vi "Volume data viewer tool.vi"() -> ()   [LabVIEW 2017]
uses:
  <vilib>/addons/Biomedical/NI_BMTK_Controls.lvlib
  <vilib>/addons/Biomedical/Controls/Medical Image/Medical Image 2D Viewer Helper (2D U16).vi
  Typedefs/Save-Load enum.ctl
  <vilib>/addons/Biomedical/Controls/Medical Image/2D Image Viewer/Medical Image 2D Viewer.xctl
panel:
  out "2D Viewer":i32[][][](xcontrol)
  in  "Selected Plane":i32(slide) scale=1.0..5.0
  in  "TDMS file path & name":path=path "C:/Users/Theo/Desktop/Volume Acquisition/Volume acquisition TDMS data files/001.tdms"
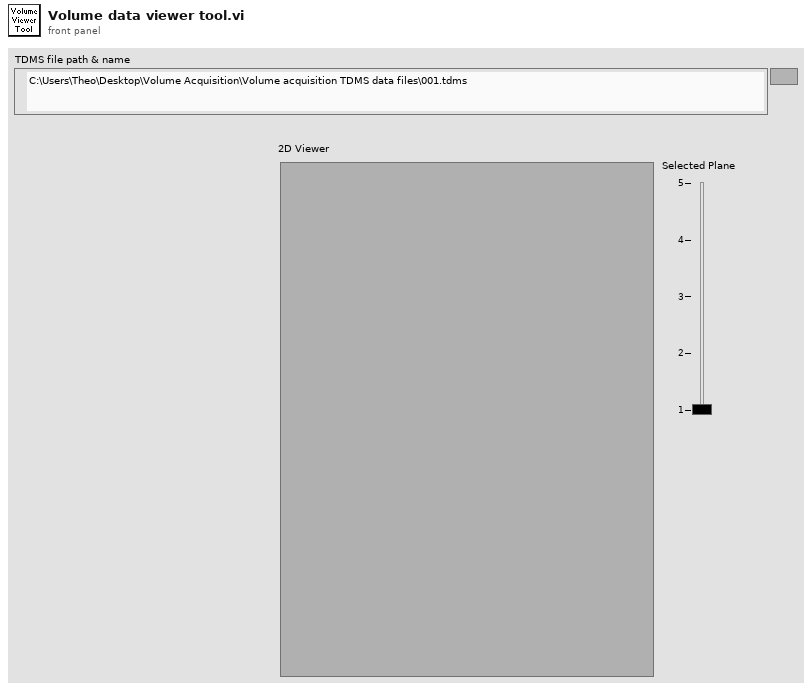
[diagram p1: front panel]
types:
  T1 = typedef "Save-Load enum.ctl" = enum16{"Save to file", "Load from file", "Compare from file"}
  T2 = typedef "Header parameters cluster-ALL.ctl" = cluster{"Imaging Protocol":T3, "Number of POI":u16, "Number of Miniscans":u16, "Number of Trials":u16, "Number of Cycles ":u64, "# Averaged Frames":u16, "Laser power (%)":u8, "Pockels":dbl, "Acquisition Length (sec)":dbl, "Fill time (us)":dbl, "POI Dwell time (us)":dbl, "Miniscan Dwell time per pixel (us)":dbl, "PMT 1":dbl, "PMT 2":dbl, "Back Apperture":dbl, "Zoom":dbl, "Frame Size":T4, "Center Frequency":dbl, "Field of View":dbl, "DwellTime (us)":dbl, "Wavelength (nm)":dbl, "AOL Z":dbl, "AOL Mode":T5, "GridXY":dbl, "GridZ":dbl, "TriggerDelay (sec)":dbl, "Number of Pixels in Miniscan":u16, "Experiment folder path":path, "X centre":dbl, "Y centre":dbl, "Angle (degrees)":dbl, "Plane Mode":T6, "Software version":dbl, "Objective":T7, "MotorZ Calibration":u32, "Pockels Calibration":u32, "Threshold":u16[], "Video length (sec)":dbl, "Frame rate (fps)":u8, "Rectangle ROI length (pixels)":u16, "Rectangle ROI height (pixels)":u16}
  T3 = typedef "Imaging Protocols enum.ctl" = enum16{"AOL Z-Stack", "Motor Z Stack", "Functional Acquisition", "Single Plane Acquisition", "Volume Acquisition", "Live Imaging", "Live Plane Imaging", "Live Volume Imaging"}
  T4 = typedef "Frame Size.ctl" = u16
  T5 = typedef "AOL modes.ctl" = enum16{"Raster", "Structural", "Pointing", "Mini Scan", "Alignment"}
  T6 = typedef "Plane Mode.ctl" = u16
  T7 = typedef "Objective selector control enum.ctl" = string
  T8 = cluster{"Number of cycles":i32, "number of planes":i32, "number of miniscans in a Plane":i32, "number of pixels in a miniscan":i32}
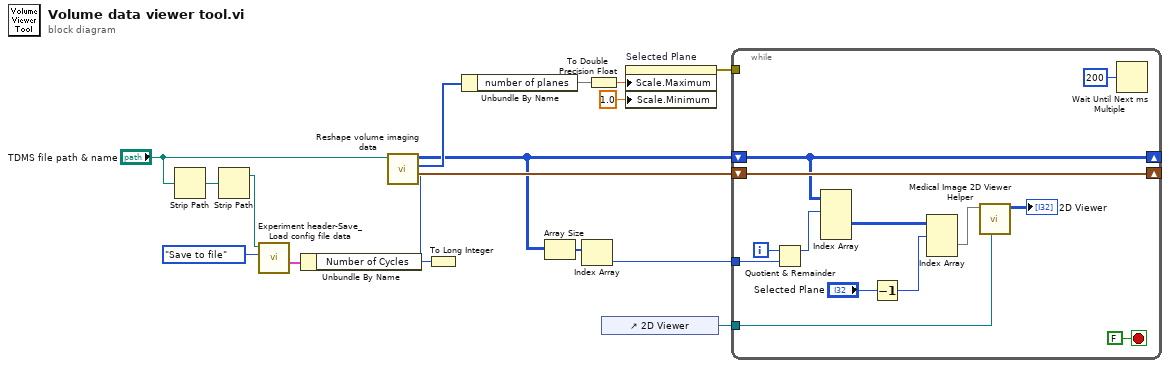
[diagram p0: block diagram]
diagram:
  n1 = Strip Path(path="TDMS file path & name") -> (stripped path=w5:path)  [unwired: 1 out]
  n2 = Strip Path(path=w5) -> (stripped path=w3:path)  [unwired: 1 out]
  n3 = call "Experiment header-Save_Load config file data.vi"("Function"=Save-Load_enum."Save to file", "Experiment data folder path"=w3) -> ("All header parameters out"=w6:T2)  [unwired: 8 in, 1 out]
  n4 = Unbundle By Name(w6) -> ("Number of Cycles"=w2:u64)
  n5 = To Long Integer(number=w2) -> (32bit integer=w1:i32)
  n6 = call "Reshape volume imaging data.vi"(9:w1, "TDMS file path & name"="TDMS file path & name") -> ("Volumetric parameters"=w9:T8, "Single channel data"=w10:u16[], "Channel 4D data"=w8:u16[][][][])  [unwired: 4 in, 3 out]
  n7 = Unbundle By Name(w10) -> ("number of planes"=w15)
  n8 = Array Size(array=w8) -> (size(s)=w17:i32[])
  n9 = Index Array(array=w17) -> (element=w16:i32)  [unwired: 1 in]
  n10 = To Double Precision Float(number=w15) -> (double precision float=w11:dbl)
  n11 = control-ref of="2D Viewer"() -> (w13:refnum<vi>)
  n12 = property on="Selected Plane" class="Slide (strict)"("Scale.Maximum"=w11, "Scale.Minimum"=1.0 ("Scale.Range:Minimum")) -> (error out=w12:errorcluster)  [unwired: 2 in, 1 out]
  n13 = while {
    shift-right: [w25] -> _
    shift-left: w8 -> [w25]
    shift-right: [w28] -> _
    shift-left: w9 -> [w28]
    tunnel: w16 -> [w27]
    tunnel: w13 -> [w19]
    tunnel: w12 -> [_]
    i -> [w26]
    stop <- FALSE stop-if-true
    n14 = Quotient & Remainder(x=w26, y=w27) -> (x-y*floor(x/y)=w24:i32)  [unwired: 1 out]
    n15 = Index Array(array=w25, index (dim 0)=w24) -> (element=w20:u16[][][])  [unwired: 3 in]
    n16 = Decrement(x="Selected Plane") -> (x-1=w22:i32)
    n17 = Index Array(array=w20, index (dim 0)=w22) -> (element=w18:u16[][])  [unwired: 2 in]
    n18 = call-poly <vilib>:"Medical Image 2D Viewer Helper.vi"("2D Viewer"=w19, "2D array in"=w18) -> ("3D array out"=→"2D Viewer":i32[][][])  [unwired: 8 in, 1 out]
    n19 = Wait Until Next ms Multiple(millisecond multiple=u32 200) -> ()  [unwired: 1 out]
  }
